vi "Setup.vi"(8 "error in (no error)":errorcluster, 9 "Amps":dbl, 10 "Volts":dbl, 11 "Power Supply in":refnum<class "Power Supply.lvclass">) -> (0 "error out":errorcluster, 3 "Power Supply out":refnum<class "Power Supply.lvclass">)   [LabVIEW 2020, in "Power Supply.lvlib" / "Power Supply.lvclass"]
uses:
  Power Supply.lvclass
  Power Supply.lvclass/Power Supply.ctl
  Write Current.vi
  Write Volts.vi
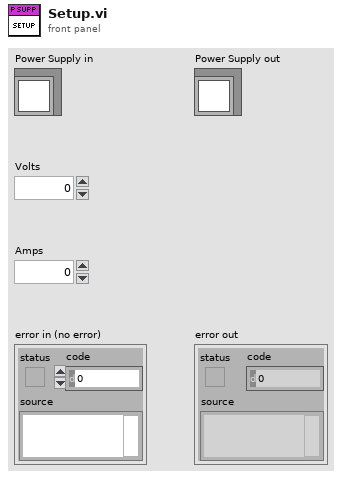
[diagram p1: front panel]
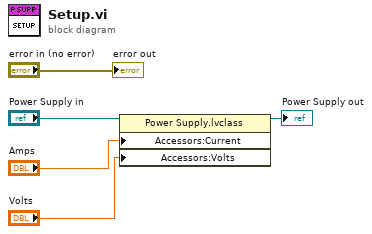
[diagram p0: block diagram]
diagram:
  n1 = property class="Power Supply.lvclass"(reference="Power Supply in", "Accessors:Current"="Amps", "Accessors:Volts"="Volts") -> (reference out=→"Power Supply out":refnum<class "Power Supply.lvclass">)  [unwired: 1 in, 1 out]
  "error out" <- "error in (no error)"
